vi "C_code.vi"(4 "Ball Diameter":i32=11, 5 "working directory":path=path "", 6 "Blue BG":T1={"Rmin"=39, "Rmax"=62, "Gmin"=91, "Gmax"=116, "Bmin"=202, "Bmax"=255}, 7 "Frame borders":T2, 8 "error in (no error)":errorcluster, 9 "White Ball":T1={"Rmin"=100, "Rmax"=255, "Gmin"=100, "Gmax"=255, "Bmin"=100, "Bmax"=255}, 10 "Yellow Ball":T1={"Rmin"=140, "Rmax"=255, "Gmin"=140, "Gmax"=255, "Bmin"=0, "Bmax"=175}, 11 "Red Ball":T1={"Rmin"=160, "Rmax"=255, "Gmin"=0, "Gmax"=160, "Bmin"=0, "Bmax"=160}) -> (0 "error out":errorcluster)   [LabVIEW 2019]
doc: "Ce VI fait appel à notre code C.\nIl prend en entrée : \n- Le cluster “Frame borders” généré par le VI “Billard borders”.\n- Les clusters “Red Ball”, “Yellow Ball”, “White ball”, “Blue BG” contenant les ranges de couleurs pour le rouge, jaune, blanc et bleu clair (couleur du tapis) respectivement.\n- Le chemin du dossier où se trouve notre VI principal “Billard2020” et le fichier “Pixmap.bin”.\n- Le diamètre de la balle (un entier)\n\nL'exécution de ce VI permet de créer un fichier “Pos.txt” dans le dossier principal (en faisant appel au code C). Le fichier “Pos.txt” contient les coordonnées des boules de chaque couleur (en pixels)."
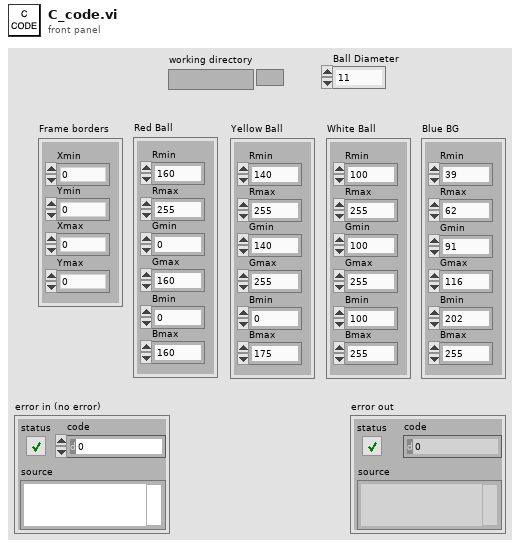
[diagram p1: front panel]
types:
  T1 = cluster{"Rmin":i32, "Rmax":i32, "Gmin":i32, "Gmax":i32, "Bmin":i32, "Bmax":i32}
  T2 = cluster{"Xmin":i32, "Ymin":i32, "Xmax":i32, "Ymax":i32}
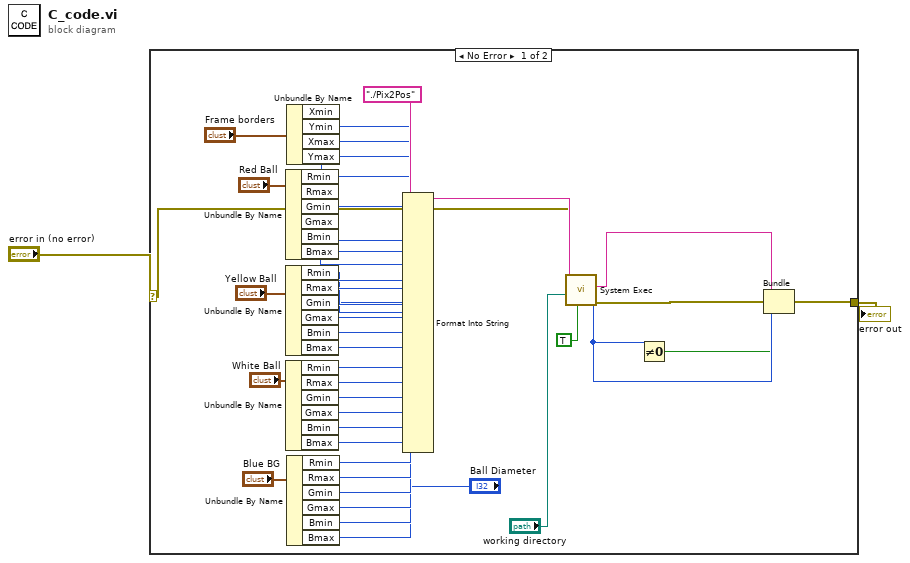
[diagram p0: block diagram]
diagram:
  n1 = case shown="No Error" "error in (no error)" {
    selector: "error in (no error)" -> [w10 w48]
    tunnel: [w6 w48] -> w1
    frame No Error {
      n2 = Unbundle By Name("Red Ball") -> ("Rmin"=w37:i32, "Rmax"=w36:i32, "Gmin"=w35:i32, "Gmax"=w34:i32, "Bmin"=w33:i32, "Bmax"=w32:i32)
      n3 = Unbundle By Name("Yellow Ball") -> ("Rmin"=w31:i32, "Rmax"=w30:i32, "Gmin"=w29:i32, "Gmax"=w28:i32, "Bmin"=w27:i32, "Bmax"=w26:i32)
      n4 = Unbundle By Name("White Ball") -> ("Rmin"=w25:i32, "Rmax"=w24:i32, "Gmin"=w23:i32, "Gmax"=w22:i32, "Bmin"=w21:i32, "Bmax"=w20:i32)
      n5 = Unbundle By Name("Frame borders") -> ("Xmin"=w39:i32, "Ymin"=w41:i32, "Xmax"=w38:i32, "Ymax"=w40:i32)
      n6 = Unbundle By Name("Blue BG") -> ("Rmin"=w19:i32, "Rmax"=w18:i32, "Gmin"=w17:i32, "Gmax"=w16:i32, "Bmin"=w15:i32, "Bmax"=w14:i32)
      n7 = Format Into String(error in=w10, "./Pix2Pos", w41, w40, w39, w38, w37, w36, w35, w34, w33, w32, w31, w30, w29, w28, w27, w26, w25, w24, w23, w22, w21, w20, w19, w18, w17, w16, w15, w14, "Ball Diameter") -> (resulting string=w12:string, error out=w9:errorcluster)  [unwired: 2 in]
      n8 = call <vilib>:"System Exec.vi"("run minimized? (F)"=TRUE, "error in (no error)"=w9, "working directory"="working directory", "command line"=w12) -> ("error out"=w5:errorcluster, "return code"=w4:i32, "standard error"=w7:string)  [unwired: 4 in, 1 out]
      n9 = Not Equal To 0?(x=w4) -> (x != 0?=w3:bool)
      n10 = Bundle(cluster=w5, "status"=w3, "code"=w4, "source"=w7) -> (w6:errorcluster)
    }
    frame Error {
    }
  }
  "error out" <- w1
